vi "Word_Set_Paragraph_Format(adv).vi"(0 "Range in":refnum<k7>, 1 "Indent and spacing":T2 {"At" format="%.2f"; "After" format="%.2f"; "Before" format="%.2f"; "By" format="%.2f"; "Right" format="%.2f"; "Left" format="%.2f"}, 2 "measurement system":u16(ring) caption="measurement system (US)", 11 "Error in":errorcluster, 12 "Line and page breaks":T3 {"Don't hyphenate" items=["Unchanged", "No", "Yes"]; "Suppress line numbers" items=["Unchanged", "No", "Yes"]; "Page break before" items=["Unchanged", "No", "Yes"]; "Keep with next" items=["Unchanged", "No", "Yes"]; "Keeps lines together" items=["Unchanged", "No", "Yes"]; "Widow/orphan ctrl" items=["Unchanged", "No", "Yes"]}) -> (4 "Range out":refnum<k7>, 15 "Error out":errorcluster)   [LabVIEW 2020, in "NI_ReportGenerationToolkit.lvlib"]
uses:
  <vilib>/addons/_office/NI_ReportGenerationToolkit.lvlib
panel:
  in  "Tab Control":T1(tab)
  # "Indentation"
  # "Spacing"
  # "Pagination"
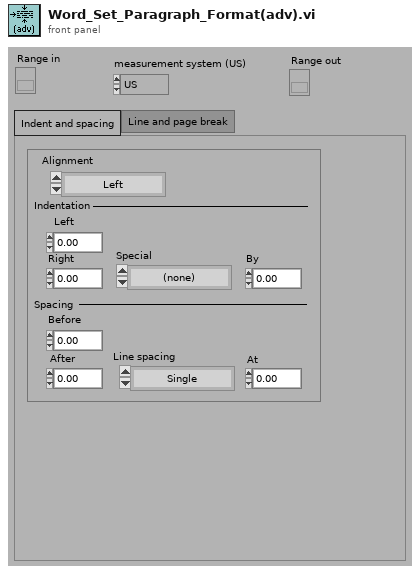
[diagram p1: front panel]
types:
  T1 = enum32{"Indent and spacing", "Line and page break"}
  T2 = cluster{"Alignment":enum16{"Left", "Centered", "Right", "Justify"}, "Left":dbl, "Right":dbl, "Special":enum16{"(none)", "First line", "Hanging"}, "By":dbl, "Before":dbl, "After":dbl, "Line spacing":enum16{"Single", "1,5 lines", "Double", "At least", "Exactly", "Multiple"}, "At":dbl}
  T3 = cluster{"Widow/orphan ctrl":u16, "Keeps lines together":u16, "Keep with next":u16, "Page break before":u16, "Suppress line numbers":u16, "Don't hyphenate":u16}
  T4 = enum16{"Single", "1,5 lines", "Double", "At least", "Exactly", "Multiple"}
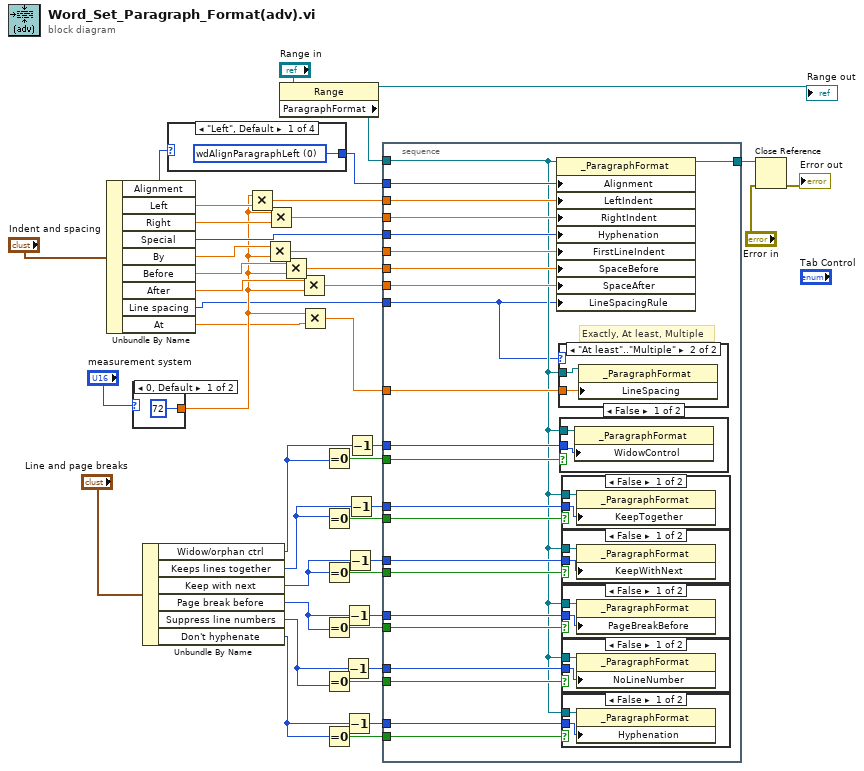
[diagram p0: block diagram]
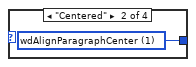
[diagram p2: hidden frame]
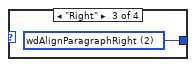
[diagram p3: hidden frame]
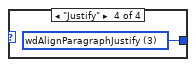
[diagram p4: hidden frame]
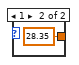
[diagram p5: hidden frame]
diagram:
  n1 = Unbundle By Name("Indent and spacing") -> ("Alignment"=w5:enum16{"Left", "Centered", "Right", "Justify"}, "Left"=w38:dbl, "Right"=w37:dbl, "Special"=w35:enum16{"(none)", "First line", "Hanging"}, "By"=w36:dbl, "Before"=w40:dbl, "After"=w39:dbl, "Line spacing"=w2:T4, "At"=w1:dbl)
  n2 = case shown="0, Default" "measurement system" {
    tunnel: [72 28.35] -> w6
    frame 0, Default {
    }
    frame 1 {
    }
  }
  n3 = Unbundle By Name("Line and page breaks") -> ("Widow/orphan ctrl"=w17:u16, "Keeps lines together"=w19:u16, "Keep with next"=w21:u16, "Page break before"=w23:u16, "Suppress line numbers"=w25:u16, "Don't hyphenate"=w28:u16)
  n4 = case shown="\"Left\", Default" w5 {
    tunnel: [w47 w48 w49 w50] -> w4
    frame "Left", Default {
      w47 = 0 items=["wdAlignParagraphLeft"=0, "wdAlignParagraphCenter"=1, "wdAlignParagraphRight"=2, "wdAlignParagraphJustify"=3, "wdAlignParagraphDistribute"=4, "wdAlignParagraphJustifyMed"=5, "wdAlignParagraphJustifyHi"=7, "wdAlignParagraphJustifyLow"=8] ("Alignment")
    }
    frame "Centered" {
      w48 = 1 items=["wdAlignParagraphLeft"=0, "wdAlignParagraphCenter"=1, "wdAlignParagraphRight"=2, "wdAlignParagraphJustify"=3, "wdAlignParagraphDistribute"=4, "wdAlignParagraphJustifyMed"=5, "wdAlignParagraphJustifyHi"=7, "wdAlignParagraphJustifyLow"=8] ("Alignment")
    }
    frame "Right" {
      w49 = 2 items=["wdAlignParagraphLeft"=0, "wdAlignParagraphCenter"=1, "wdAlignParagraphRight"=2, "wdAlignParagraphJustify"=3, "wdAlignParagraphDistribute"=4, "wdAlignParagraphJustifyMed"=5, "wdAlignParagraphJustifyHi"=7, "wdAlignParagraphJustifyLow"=8] ("Alignment")
    }
    frame "Justify" {
      w50 = 3 items=["wdAlignParagraphLeft"=0, "wdAlignParagraphCenter"=1, "wdAlignParagraphRight"=2, "wdAlignParagraphJustify"=3, "wdAlignParagraphDistribute"=4, "wdAlignParagraphJustifyMed"=5, "wdAlignParagraphJustifyHi"=7, "wdAlignParagraphJustifyLow"=8] ("Alignment")
    }
  }
  n5 = Multiply(x=w6, y=w38) -> (x*y=w12:dbl)
  n6 = Multiply(x=w36, y=w6) -> (x*y=w10:dbl)
  n7 = Multiply(x=w6, y=w37) -> (x*y=w11:dbl)
  n8 = property class="Range"(reference="Range in") -> (reference out=→"Range out":refnum<k7>, "ParagraphFormat"=w16:refnum<k7>)  [unwired: 1 in, 1 out]
  n9 = Multiply(x=w40, y=w6) -> (x*y=w9:dbl)
  n10 = Multiply(x=w39, y=w6) -> (x*y=w8:dbl)
  n11 = Multiply(x=w6, y=w1) -> (x*y=w7:dbl)
  n12 = Equal To 0?(x=w17) -> (x = 0?=w29:bool)
  n13 = Equal To 0?(x=w19) -> (x = 0?=w34:bool)
  n14 = Equal To 0?(x=w21) -> (x = 0?=w33:bool)
  n15 = Equal To 0?(x=w23) -> (x = 0?=w32:bool)
  n16 = Equal To 0?(x=w25) -> (x = 0?=w31:bool)
  n17 = Equal To 0?(x=w28) -> (x = 0?=w30:bool)
  n18 = Decrement(x=w25) -> (x-1=w26:u16)
  n19 = Decrement(x=w23) -> (x-1=w24:u16)
  n20 = Decrement(x=w28) -> (x-1=w27:u16)
  n21 = Decrement(x=w21) -> (x-1=w22:u16)
  n22 = Decrement(x=w19) -> (x-1=w20:u16)
  n23 = Decrement(x=w17) -> (x-1=w18:u16)
  n24 = stacked-sequence {
    tunnel: w7 -> [w53]
    tunnel: w2 -> [w51]
    tunnel: w9 -> [w73]
    tunnel: w8 -> [w72]
    tunnel: w4 -> [w71]
    tunnel: w12 -> [w70]
    tunnel: w11 -> [w69]
    tunnel: w10 -> [w68]
    tunnel: w35 -> [w67]
    tunnel: w34 -> [w66]
    tunnel: w33 -> [w65]
    tunnel: w32 -> [w64]
    tunnel: w31 -> [w63]
    tunnel: w30 -> [w62]
    tunnel: w29 -> [w61]
    tunnel: w27 -> [w60]
    tunnel: w26 -> [w59]
    tunnel: w24 -> [w58]
    tunnel: w22 -> [w57]
    tunnel: w20 -> [w56]
    tunnel: w18 -> [w55]
    tunnel: w16 -> [w52]
    tunnel: [w54] -> w15
    frame #0 {
      # "Exactly, At least, Multiple"
      n25 = property class="_ParagraphFormat"(reference=w52, "Alignment"=w71, "LeftIndent"=w70, "RightIndent"=w69, "Hyphenation"=w67, "FirstLineIndent"=w68, "SpaceBefore"=w73, "SpaceAfter"=w72, "LineSpacingRule"=w51) -> (reference out=w54:refnum<k7>)  [unwired: 1 in, 1 out]
      n26 = case shown="\"At least\"..\"Multiple\"" w51 {
        tunnel: w53 -> [_ w75]
        tunnel: w52 -> [_ w74]
        frame Default {
        }
        frame "At least".."Multiple" {
          n27 = property class="_ParagraphFormat"(reference=w74, "LineSpacing"=w75) -> ()  [unwired: 1 in, 2 out]
        }
      }
      n28 = case shown="False" w61 {
        tunnel: w55 -> [w87 _]
        tunnel: w52 -> [w86 _]
        frame False {
          n29 = property class="_ParagraphFormat"(reference=w86, "WidowControl"=w87) -> ()  [unwired: 1 in, 2 out]
        }
        frame True {
        }
      }
      n30 = case shown="False" w66 {
        tunnel: w56 -> [w85 _]
        tunnel: w52 -> [w84 _]
        frame False {
          n31 = property class="_ParagraphFormat"(reference=w84, "KeepTogether"=w85) -> ()  [unwired: 1 in, 2 out]
        }
        frame True {
        }
      }
      n32 = case shown="False" w65 {
        tunnel: w57 -> [w83 _]
        tunnel: w52 -> [w82 _]
        frame False {
          n33 = property class="_ParagraphFormat"(reference=w82, "KeepWithNext"=w83) -> ()  [unwired: 1 in, 2 out]
        }
        frame True {
        }
      }
      n34 = case shown="False" w64 {
        tunnel: w58 -> [w81 _]
        tunnel: w52 -> [w80 _]
        frame False {
          n35 = property class="_ParagraphFormat"(reference=w80, "PageBreakBefore"=w81) -> ()  [unwired: 1 in, 2 out]
        }
        frame True {
        }
      }
      n36 = case shown="False" w63 {
        tunnel: w59 -> [w79 _]
        tunnel: w52 -> [w78 _]
        frame False {
          n37 = property class="_ParagraphFormat"(reference=w78, "NoLineNumber"=w79) -> ()  [unwired: 1 in, 2 out]
        }
        frame True {
        }
      }
      n38 = case shown="False" w62 {
        tunnel: w60 -> [w77 _]
        tunnel: w52 -> [w76 _]
        frame False {
          n39 = property class="_ParagraphFormat"(reference=w76, "Hyphenation"=w77) -> ()  [unwired: 1 in, 2 out]
        }
        frame True {
        }
      }
    }
  }
  n40 = Close Reference(reference=w15, error in (no error)="Error in") -> (error out=→"Error out":errorcluster)
